vi "Gaussians with offset with cov cor.vi"(9 "initial guess":T2={"initial amplitude"=645096.1306995839, "initial center"=3.6928451722104705, "initial standard deviation"=0.1, "offset"=100.0}, 10 "X":dbl[](array[numeric])=[3.586800426606236, 3.590013903745758, 3.5932273808852804, 3.5964408580248026, 3.599654335164325, 3.602867812303847, 3.6060812894433694, 3.6092947665828916, 3.612508243722414, 3.615721720861936, 3.6189351980014584, 3.6221486751409806, 3.625362152280503, 3.6285756294200255, 3.631789106559548, 3.63500258369907, 3.6382160608385923, 3.6414295379781145, 3.6446430151176368, 3.647856492257159, 3.6510699693966813, 3.6542834465362035, 3.6574969236757258, 3.660710400815248, 3.6639238779547703, 3.6671373550942925, 3.6703508322338148, 3.673564309373337, 3.6767777865128592, 3.6799912636523815, 3.6832047407919037, 3.686418217931426, 3.6896316950709482, 3.6928451722104705, 3.696058649349993, 3.6992721264895154, 3.7024856036290377, 3.70569908076856, 3.708912557908082, 3.7121260350476044, 3.7153395121871267, 3.718552989326649, 3.721766466466171, 3.7249799436056934, 3.7281934207452156, 3.731406897884738, 3.73462037502426, 3.7378338521637824, 3.7410473293033046, 3.744260806442827, 3.747474283582349, 3.7506877607218714, 3.7539012378613936, 3.757114715000916, 3.760328192140438, 3.763541669279961, 3.766755146419483, 3.7699686235590053, 3.7731821006985276, 3.77639557783805, 3.779609054977572, 3.7828225321170943, 3.7860360092566165, 3.789249486396139, 3.792462963535661, 3.7956764406751833, 3.7988899178147055], 11 "Y":dbl[](array[numeric])=[122471.39815898682, 136410.14855397973, 148935.28860990095, 163320.20150307816, 178749.67418397317, 196938.64335096432, 213396.63485045257, 231164.5356937577, 249693.77493685717, 270458.2424419016, 289674.3811359848, 309747.60541087727, 331076.1656568719, 354057.95339389576, 375001.4704833015, 395953.11173051764, 418271.4276096431, 441600.2878281491, 462355.92865030374, 482232.4240565795, 503051.2209438647, 523748.0120689487, 542248.1675243961, 559543.972225563, 576441.2765237598, 591958.7603438987, 604887.8303387399, 615956.0190536586, 626282.7699151189, 634663.4952645759, 639937.6675845425, 643574.0107088247, 645555.6693692375, 645096.1306995839, 642436.5319770848, 638641.9402795356, 633412.4734295781, 626182.0686752424, 616795.4482366381, 606605.5657346066, 594639.8417383569, 579934.4446803913, 563707.4106605576, 547172.8184056595, 529321.3377983638, 509605.0687427654, 489331.80819200526, 469572.80876748014, 449469.6706969484, 427606.51024418604, 406478.0731453054, 386730.3927565679, 367087.1602034074, 345316.2996502439, 324940.29952309455, 306198.4721711825, 287980.7970451663, 267659.3367570957, 249272.76509165356, 231699.4458730044, 215620.60396586897, 198251.7496494042, 183483.8357103524, 169596.40766546674, 157527.0313991652, 143526.58092590055, 132183.65333496485]) -> (0 "R-square":dbl, 1 "FWHM":dbl, 2 "Parameters Fit":T1, 3 "best nonlinear fit":dbl[](array[numeric]))   [LabVIEW 2023]
uses:
  <vilib>/Analysis/Matrix/Datatypes/RealMatrix.ctl
  <vilib>/gmath/NumericalOptimization/Nonlinear Curve Fit LM.vi
  <vilib>/gmath/NI_Gmath.lvlib
  <vilib>/Analysis/Matrix/NI_Matrix.lvlib
panel:
  out "covariance":T3
  out "best fit parameters":dbl[](array[numeric])
  out "error out":errorcluster
  in  "termination":cluster{"max iteration":i32, "tolerance":dbl}={"max iteration"=200, "tolerance"=1e-08}
  out "XY Graph":cluster{"subarray 2":dbl[], "subarray":dbl[]}[](graph)
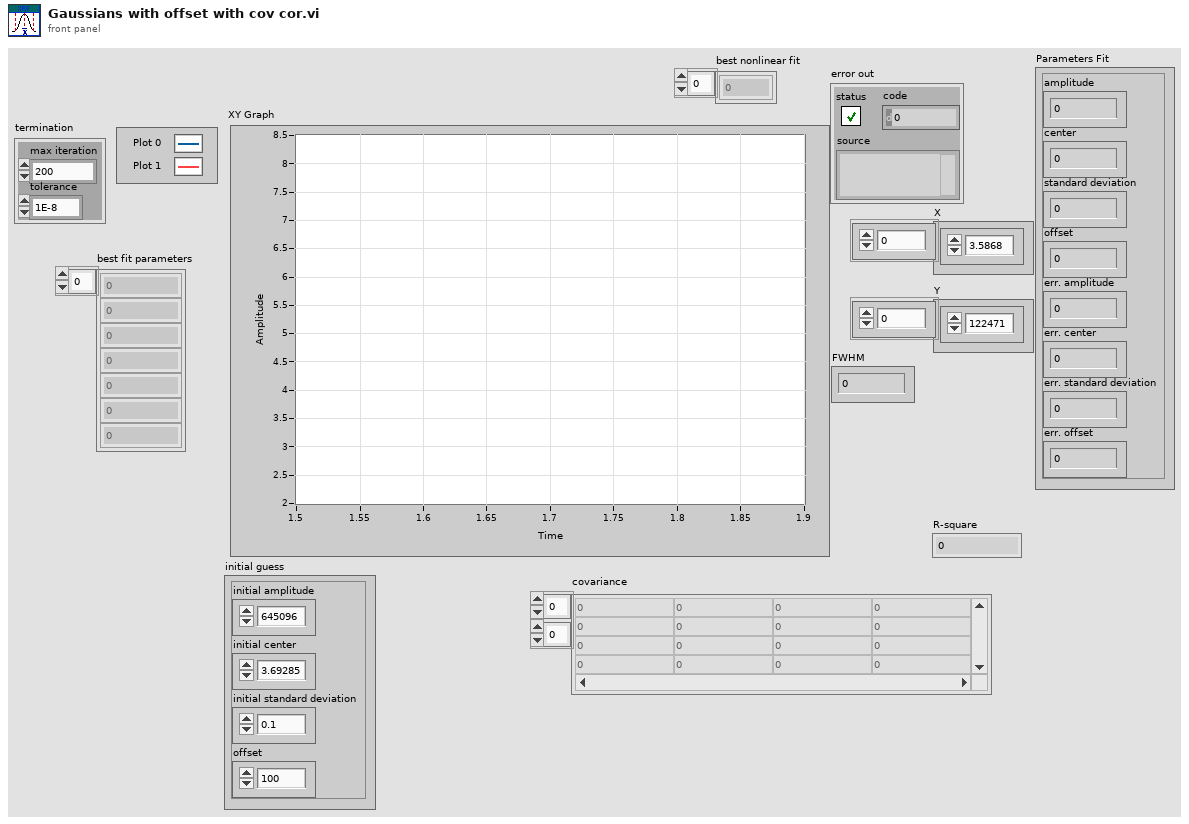
[diagram p1: front panel]
types:
  T1 = cluster{"amplitude":dbl, "center":dbl, "standard deviation":dbl, "offset":dbl, "err. amplitude":dbl, "err. center":dbl, "err. standard deviation":dbl, "err. offset":dbl}
  T2 = cluster{"initial amplitude":dbl, "initial center":dbl, "initial standard deviation":dbl, "offset":dbl}
  T3 = typedef "NI_Matrix.lvlib/RealMatrix.ctl" = dbl[][]
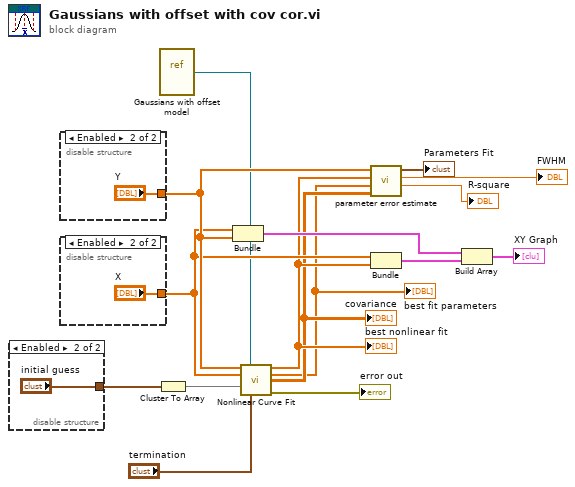
[diagram p0: block diagram]
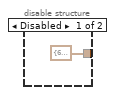
[diagram p2: hidden frame]
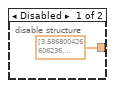
[diagram p3: hidden frame]
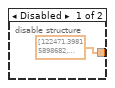
[diagram p4: hidden frame]
diagram:
  n1 = disable-structure shown="Enabled" {
    disable-tunnel: [T2 {"initial amplitude"=645096.1306995839, "initial center"=3.6928451722104705, "initial standard deviation"=0.1, "offset"=100.0} ("output cluster 2") "initial guess"] -> w16
    frame Disabled {
    }
    frame Enabled {
    }
  }
  n2 = disable-structure shown="Enabled" {
    disable-tunnel: [dbl[] [122471.39815898682, 136410.14855397973, 148935.28860990095, 163320.20150307816, 178749.67418397317, 196938.64335096432, 213396.63485045257, 231164.5356937577, 249693.77493685717, 270458.2424419016, 289674.3811359848, 309747.60541087727, 331076.1656568719, 354057.95339389576, 375001.4704833015, 395953.11173051764, 418271.4276096431, 441600.2878281491, 462355.92865030374, 482232.4240565795, 503051.2209438647, 523748.0120689487, 542248.1675243961, 559543.972225563, 576441.2765237598, 591958.7603438987, 604887.8303387399, 615956.0190536586, 626282.7699151189, 634663.4952645759, 639937.6675845425, 643574.0107088247, 645555.6693692375, 645096.1306995839, 642436.5319770848, 638641.9402795356, 633412.4734295781, 626182.0686752424, 616795.4482366381, 606605.5657346066, 594639.8417383569, 579934.4446803913, 563707.4106605576, 547172.8184056595, 529321.3377983638, 509605.0687427654, 489331.80819200526, 469572.80876748014, 449469.6706969484, 427606.51024418604, 406478.0731453054, 386730.3927565679, 367087.1602034074, 345316.2996502439, 324940.29952309455, 306198.4721711825, 287980.7970451663, 267659.3367570957, 249272.76509165356, 231699.4458730044, 215620.60396586897, 198251.7496494042, 183483.8357103524, 169596.40766546674, 157527.0313991652, 143526.58092590055, 132183.65333496485] ("subarray") "Y"] -> w9
    frame Disabled {
    }
    frame Enabled {
    }
  }
  n3 = disable-structure shown="Enabled" {
    disable-tunnel: [dbl[] [3.586800426606236, 3.590013903745758, 3.5932273808852804, 3.5964408580248026, 3.599654335164325, 3.602867812303847, 3.6060812894433694, 3.6092947665828916, 3.612508243722414, 3.615721720861936, 3.6189351980014584, 3.6221486751409806, 3.625362152280503, 3.6285756294200255, 3.631789106559548, 3.63500258369907, 3.6382160608385923, 3.6414295379781145, 3.6446430151176368, 3.647856492257159, 3.6510699693966813, 3.6542834465362035, 3.6574969236757258, 3.660710400815248, 3.6639238779547703, 3.6671373550942925, 3.6703508322338148, 3.673564309373337, 3.6767777865128592, 3.6799912636523815, 3.6832047407919037, 3.686418217931426, 3.6896316950709482, 3.6928451722104705, 3.696058649349993, 3.6992721264895154, 3.7024856036290377, 3.70569908076856, 3.708912557908082, 3.7121260350476044, 3.7153395121871267, 3.718552989326649, 3.721766466466171, 3.7249799436056934, 3.7281934207452156, 3.731406897884738, 3.73462037502426, 3.7378338521637824, 3.7410473293033046, 3.744260806442827, 3.747474283582349, 3.7506877607218714, 3.7539012378613936, 3.757114715000916, 3.760328192140438, 3.763541669279961, 3.766755146419483, 3.7699686235590053, 3.7731821006985276, 3.77639557783805, 3.779609054977572, 3.7828225321170943, 3.7860360092566165, 3.789249486396139, 3.792462963535661, 3.7956764406751833, 3.7988899178147055] ("subarray 2") "X"] -> w8
    frame Disabled {
    }
    frame Enabled {
    }
  }
  n4 = Cluster To Array(cluster=w16) -> (array=w15:dbl[])
  n5 = vi-ref "Gaussians with offset model.vi"() -> (w1:refnum<vi>)
  n6 = Bundle("X"=w8, "Y"=w9) -> (w11:cluster{"X":dbl[], "Y":dbl[]})  [unwired: 1 in]
  n7 = call-poly <vilib>:"Nonlinear Curve Fit.vi"("Y"=w9, "f(x,a)"=w1, "X"=w8, "initial parameters"=w15, "termination"="termination") -> ("best nonlinear fit"=w7:dbl[], "best fit parameters"=w5:dbl[], "covariance"=w6:T3, "error out"=→"error out":errorcluster)  [unwired: 5 in, 2 out]
  "best fit parameters" <- w5
  "covariance" <- w6
  "best nonlinear fit" <- w7
  n8 = call "parameter error estimate.vi"("covariance"=w6, "best fit parameters"=w5, "best nonlinear fit"=w7, "Y"=w9) -> ("R-square"=→"R-square":dbl, "FWHM"=→"FWHM":dbl, "Parameters Fit"=→"Parameters Fit":T1)  [unwired: 5 in]
  n9 = Bundle("X"=w8, "best nonlinear fit"=w7) -> (w10:cluster{"X":dbl[], "best nonlinear fit":dbl[]})  [unwired: 1 in]
  n10 = Build Array(w11, w10) -> (→"XY Graph":cluster{"X":dbl[], "best nonlinear fit":dbl[]}[])
